vi "Process.vi"(0 "Process In":refnum<class "Process.lvclass">, 11 "Error In":errorcluster) -> (4 "Process Out":refnum<class "Process.lvclass">, 15 "Error Out":errorcluster)   [LabVIEW 2023, in "Process.lvclass"]
doc: "Process VI that defines what specific process can do in form of state machine."
uses:
  Process.lvclass
  Private/Ctrls/Process Variables.ctl
  Interfaces/ICanCommunicate/Message.ctl
  Process.lvclass/Process.ctl
  Interfaces/ICanCommunicate/ICanCommunicate.lvclass
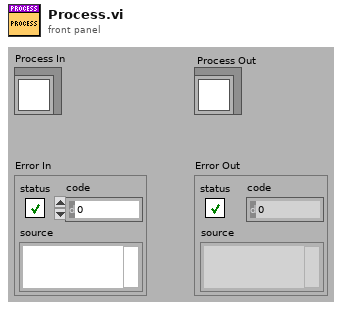
[diagram p1: front panel]
types:
  T1 = typedef "ICanCommunicate.lvclass/Message.ctl" = cluster{"Sender Name":string, "Recipent Name":string, "Command":string, "Data":variant, "Time Stamp":timestamp, "GUID":string, "Chcecksum":string}
  T2 = typedef "Process.lvclass/Process Variables.ctl" = cluster{"Local Variable":string}
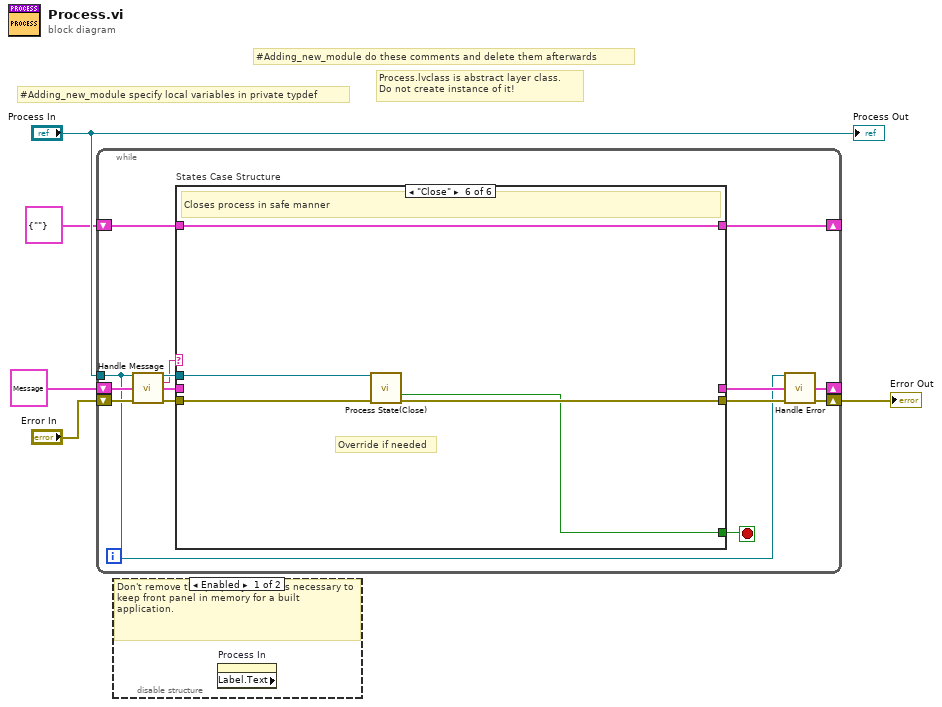
[diagram p0: block diagram]
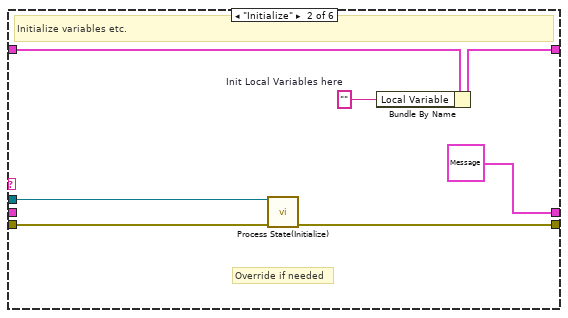
[diagram p4: hidden frame]
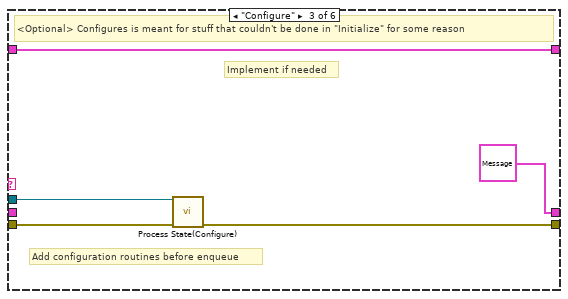
[diagram p5: hidden frame]
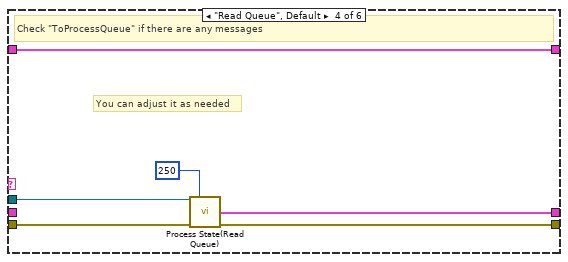
[diagram p6: hidden frame]
diagram:
  # "#Adding_new_module do these comments and delete them afterwards"
  # "#Adding_new_module specify local variables in private typdef"
  # "Process.lvclass is abstract layer class. \nDo not create instance of it!"
  n1 = while {
    shift-right: [w9] -> w5
    shift-left: "Error In" -> [w15]
    tunnel: "Process In" -> [w6]
    shift-right: [w18] -> _
    shift-left: T2 {"Local Variable"=""} ("Process Variables") -> [w17]
    shift-right: [w7] -> _
    shift-left: T1 {"Sender Name"="", "Recipent Name"="", "Command"="Initialize", "Data"=variant, "Time Stamp"=timestamp(0 s since 1904-01-01), "GUID"="", "Chcecksum"=""} ("Message") -> [w12]
    stop <- w16 stop-if-true
    n2 = call-dynamic "Handle Message.vi"("ICanComunicate In"=w6, "Message In"=w12, "Error In"=w15) -> ("ICanComunicate Out"=w11:refnum<class "Process.lvclass">, "CMD Out"=w10:string, "Message Out"=w13:T1, "Error Out"=w14:errorcluster)  [unwired: 9 in]
    n3 = case "States Case Structure" shown="\"Close\"" w10 {
      tunnel: w14 -> [w22 w27 w31 w39 w43 w47]
      tunnel: [w22 w24 w30 w38 w43 w45] -> w19
      tunnel: [w21 w29 w34 w40 w42 w48] -> w18
      tunnel: w17 -> [w21 w26 w34 w40 w42 w48]
      tunnel: [_ _ _ _ _ w44] -> w16
      tunnel: w13 -> [w20 _ _ _ w41 _]
      tunnel: [w20 T1 {"Sender Name"="", "Recipent Name"="", "Command"="Read Queue", "Data"=variant, "Time Stamp"=timestamp(0 s since 1904-01-01), "GUID"="", "Chcecksum"=""} ("Message") T1 {"Sender Name"="", "Recipent Name"="", "Command"="Read Queue", "Data"=variant, "Time Stamp"=timestamp(0 s since 1904-01-01), "GUID"="", "Chcecksum"=""} ("Message") w37 w41 _] -> w8
      tunnel: w11 -> [_ w23 w32 w36 _ w46]
      frame "--- Common ---" {
        # "Only for grouping"
      }
      frame "Initialize" {
        w28 = ""  # Init Local Variables here
        # "Override if needed"
        # "Initialize variables etc."
        n4 = call-dynamic "Process State(Initialize).vi"("Process In"=w23, "Error In"=w27) -> ("Error Out"=w24:errorcluster)  [unwired: 12 in, 1 out]
        n5 = Bundle By Name(cluster=w26, "Local Variable"=w28) -> (w29:T2)
      }
      frame "Configure" {
        # "Implement if needed"
        # "Add configuration routines before enqueue"
        # "<Optional> Configures is meant for stuff that couldn't be done in \"Initialize\" for some reason"
        n6 = call-dynamic "Process State(Configure).vi"("Process In"=w32, "Error In"=w31) -> ("Error Out"=w30:errorcluster)  [unwired: 12 in, 1 out]
      }
      frame "Read Queue", Default {
        # "You can adjust it as needed"
        # "Check \"ToProcessQueue\" if there are any messages"
        n7 = call-dynamic "Process State(Read Queue).vi"("Process In"=w36, "Timeout in ms (-1)"=250, "Error In"=w39) -> ("Message"=w37:T1, "Error Out"=w38:errorcluster)  [unwired: 9 in, 2 out]
      }
      frame "Timeout" {
        # "<Optional> Actions to be taken if there are no messages for process"
      }
      frame "Close" {
        # "Override if needed"
        # "Closes process in safe manner"
        n8 = call-dynamic "Process State(Close).vi"("Process In"=w46, "Error In"=w47) -> ("Close?"=w44:bool, "Error Out"=w45:errorcluster)  [unwired: 11 in, 1 out]
      }
    }
    n9 = call-dynamic "Handle Error.vi"("Process In"=w6, "Message In"=w8, "Error In"=w19) -> ("Message Out"=w7:T1, "Error Out"=w9:errorcluster)  [unwired: 10 in, 1 out]
  }
  "Error Out" <- w5
  n10 = disable-structure shown="Enabled" {
    frame Enabled {
      # "Don't remove this property node it's necessary to keep front panel in memory for a built application."
      n11 = property on="Process In" class="LVClassControl (strict)" props=["Label", "Text"]() -> ()  [unwired: 2 in, 3 out]
    }
    frame Disabled {
    }
  }
  "Process Out" <- "Process In"
